vi "rotate-part3.vi"(10 "Angle":i32, 11 "SceneObject输入":refnum<vi>) -> ()   [LabVIEW 2013]
uses:
  <vilib>/picture/3D Picture Control/NI_3D Picture Control.lvlib
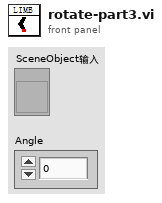
[diagram p1: front panel]
types:
  T1 = cluster{"zuoqian1":refnum<vi>, "zuoqian2":refnum<vi>, "zuoqian3":refnum<vi>}
  T2 = cluster{"youqian1":refnum<vi>, "youqian2":refnum<vi>, "youqian3":refnum<vi>}
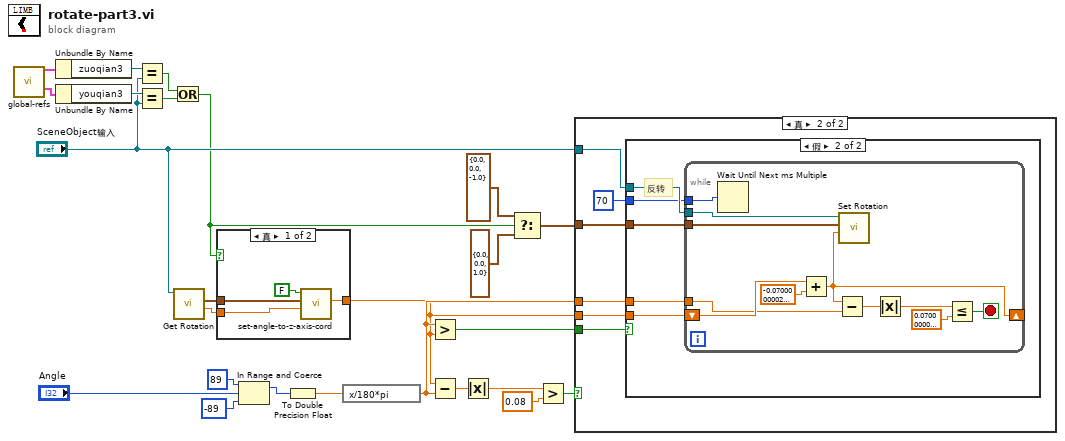
[diagram p0: block diagram]
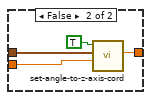
[diagram p2: hidden frame]
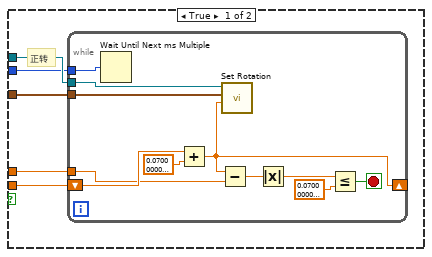
[diagram p4: hidden frame]
diagram:
  n1 = call "global-refs.vi"() -> ("ZuoQianRef"=w6:T1, "YouQianRef"=w5:T2)  [unwired: 10 in, 4 out]
  n2 = Unbundle By Name(w6) -> ("zuoqian3"=w14:refnum<vi>)
  n3 = Unbundle By Name(w5) -> ("youqian3"=w13:refnum<vi>)
  n4 = Equal?(x=w14, y="SceneObject输入") -> (x = y?=w16:bool)
  n5 = Equal?(x=w13, y="SceneObject输入") -> (x = y?=w15:bool)
  n6 = Or(x=w16, y=w15) -> (x .or. y?=w10:bool)
  n7 = call <vilib>:"Get Rotation.vi"("Scene Object"="SceneObject输入") -> ("Angle"=w8:sgl, "Axis"=w9:cluster{"X":sgl, "Y":sgl, "Z":sgl})  [unwired: 7 in, 2 out]
  n8 = case shown="真" w10 {
    tunnel: w9 -> [w28 w32]
    tunnel: w8 -> [w27 w31]
    tunnel: [w26 w30] -> w7
    frame True {
      n9 = call "set-angle-to-z-axis-cord.vi"("rad"=w27, "Axis"=w28, "正Z轴?"=FALSE) -> ("数值输入控件"=w26:dbl)  [unwired: 8 in]
    }
    frame False {
      n10 = call "set-angle-to-z-axis-cord.vi"("rad"=w31, "Axis"=w32, "正Z轴?"=TRUE) -> ("数值输入控件"=w30:dbl)  [unwired: 8 in]
    }
  }
  n11 = In Range and Coerce(upper limit=89 ("上限"), x="Angle", lower limit=-89 ("下限")) -> (coerced(x)=w2:i32)  [unwired: 1 out]
  n12 = To Double Precision Float(number=w2) -> (double precision float=w19:dbl)
  n13 = expression code="x/180*pi"(w19) -> (w24:dbl)
  n14 = Greater?(x=w24, y=w7) -> (0:w25:bool)
  n15 = Subtract(x=w7, y=w24) -> (x-y=w20:dbl)
  n16 = Absolute Value(x=w20) -> (abs(x)=w21:dbl)
  n17 = Select(t=cluster{"X":sgl, "Y":sgl, "Z":sgl} {"X"=0.0, "Y"=0.0, "Z"=-1.0} ("Axis"), s=w10, f=cluster{"X":sgl, "Y":sgl, "Z":sgl} {"X"=0.0, "Y"=0.0, "Z"=1.0} ("Axis")) -> (s? t:f=w12:cluster{"X":sgl, "Y":sgl, "Z":sgl})
  n18 = Greater?(x=w21, y=0.08) -> (0:w23:bool)
  n19 = case shown="真" w23 {
    tunnel: "SceneObject输入" -> [_ w39]
    tunnel: w24 -> [_ w35]
    tunnel: w25 -> [_ w38]
    tunnel: w12 -> [_ w37]
    tunnel: w7 -> [_ w36]
    frame False {
    }
    frame True {
      n20 = case shown="假" w38 {
        tunnel: w39 -> [w44 w60]
        tunnel: w37 -> [w43 w59]
        tunnel: w36 -> [w42 w58]
        tunnel: w35 -> [w41 w57]
        tunnel: u32 70 ("毫秒倍数") -> [w40 w56]
        frame True {
          # "正转"
          n21 = while {
            tunnel: w44 -> [w49]
            tunnel: w43 -> [w48]
            shift-right: [w46] -> _
            shift-left: w42 -> [w50]
            tunnel: w41 -> [w47]
            tunnel: w40 -> [w45]
            stop <- w51 stop-if-true
            n22 = Wait Until Next ms Multiple(millisecond multiple=w45) -> ()  [unwired: 1 out]
            n23 = Add(x=w50, y=sgl 0.07) -> (x+y=w46:dbl)
            n24 = Subtract(x=w46, y=w47) -> (x-y=w53:dbl)
            n25 = call <vilib>:"Set Rotation.vi"("Angle"=w46, "Axis"=w48, "Scene Object"=w49) -> ()  [unwired: 7 in, 2 out]
            n26 = Absolute Value(x=w53) -> (abs(x)=w54:dbl)
            n27 = Less Or Equal?(x=w54, y=sgl 0.07) -> (x <= y?=w51:bool)
          }
        }
        frame False {
          # "反转"
          n28 = while {
            tunnel: w60 -> [w65]
            tunnel: w59 -> [w64]
            shift-right: [w62] -> _
            shift-left: w58 -> [w66]
            tunnel: w57 -> [w63]
            tunnel: w56 -> [w61]
            stop <- w67 stop-if-true
            n29 = Wait Until Next ms Multiple(millisecond multiple=w61) -> ()  [unwired: 1 out]
            n30 = Add(x=w66, y=sgl -0.07) -> (x+y=w62:dbl)
            n31 = Subtract(x=w62, y=w63) -> (x-y=w69:dbl)
            n32 = call <vilib>:"Set Rotation.vi"("Angle"=w62, "Axis"=w64, "Scene Object"=w65) -> ()  [unwired: 7 in, 2 out]
            n33 = Absolute Value(x=w69) -> (abs(x)=w70:dbl)
            n34 = Less Or Equal?(x=w70, y=sgl 0.07) -> (x <= y?=w67:bool)
          }
        }
      }
    }
  }
